vi "Adjust Text to Fit Rectangle.vi"(0 "VI Name":string, 5 "Number of Rows":i32, 7 "Text settings":T1 {"Alignment" items=["left", "center", "right"]}) -> (4 "Text out":T4)   [LabVIEW 2021, in "Text-Based VI Icon.lvlib"]
uses:
  Text-Based VI Icon.lvlib
  API_Text.ctl
  API_Test Settings.ctl
  lv_icon/Controls/Alignment.ctl
  API_Text Colors.ctl
  LabVIEW Icon API.lvlib
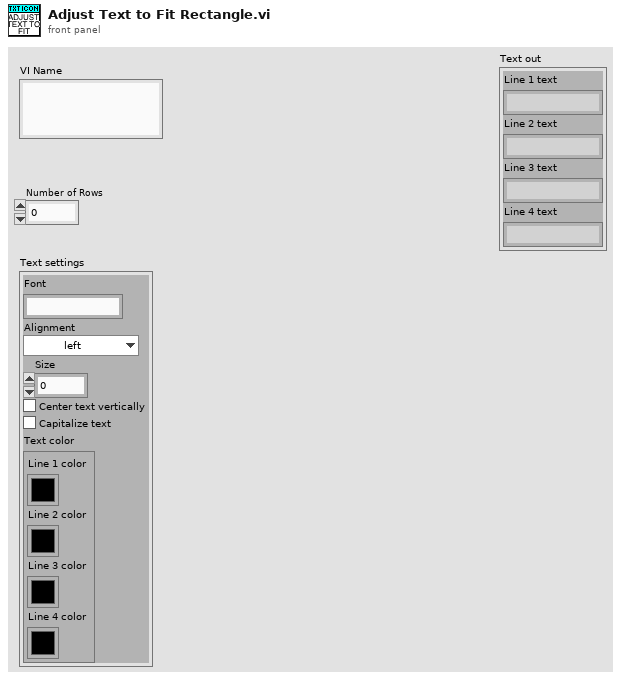
[diagram p1: front panel]
types:
  T1 = typedef "LabVIEW Icon API.lvlib/API_Test Settings.ctl" = cluster{"Font":string, "Alignment":T2, "Size":u8, "Center text":bool, "Capitalize text":bool, "Text color":T3}
  T2 = typedef "Alignment.ctl" = u16
  T3 = typedef "LabVIEW Icon API.lvlib/API_Text Colors.ctl" = cluster{"Line 1 color":u32, "Line 2 color":u32, "Line 3 color":u32, "Line 4 color":u32}
  T4 = typedef "LabVIEW Icon API.lvlib/API_Text.ctl" = cluster{"Line 1 text":string, "Line 2 text":string, "Line 3 text":string, "Line 4 text":string}
  T5 = cluster{"Font Name:":string, "Size":i16, "Strikeout?":bool, "Italic?":bool, "Underline?":bool, "Outline?":bool, "Shadow?":bool, "Bold?":bool}
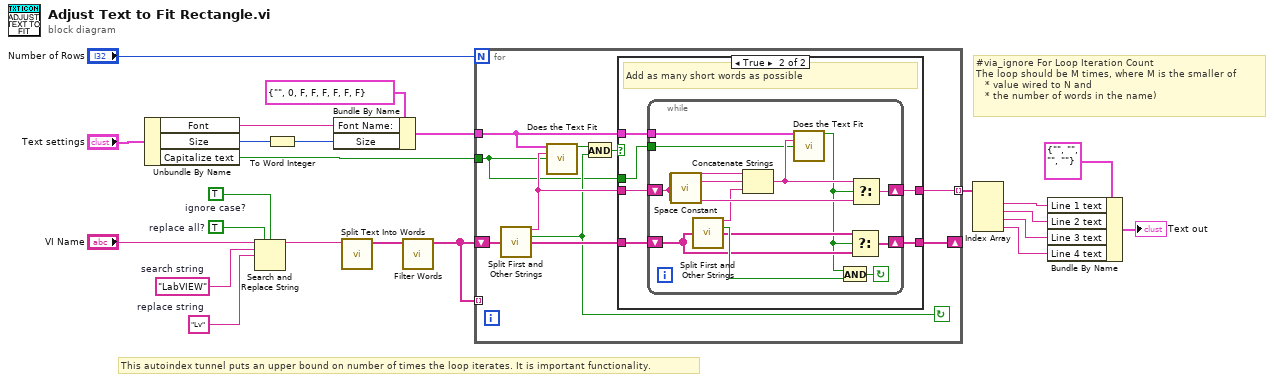
[diagram p0: block diagram]
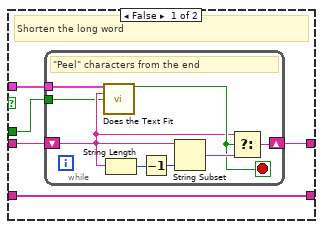
[diagram p2: hidden frame]
diagram:
  w3 = TRUE  # ignore case?
  w4 = TRUE  # replace all?
  w5 = "Lv"  # replace string
  w6 = "LabVIEW"  # search string
  # "This autoindex tunnel puts an upper bound on number of times the loop iterates. It is important functionality."
  # "#via_ignore For Loop Iteration Count\nThe loop should be M times, where M is the smaller of \n   * value wired to N and \n   * the number of words in the name)"
  n1 = Unbundle By Name("Text settings") -> ("Font"=w14:string, "Size"=w13:u8, "Capitalize text"=w9:bool)
  n2 = Search and Replace String(replace all?=w4, case sensitive?=w3, input string="VI Name", search string=w6, replace string=w5) -> (result string=w1:string)  [unwired: 3 in, 3 out]
  n3 = To Word Integer(number=w13) -> (16bit integer=w10:i16)
  n4 = Bundle By Name(cluster=T5 {"Font Name:"="", "Size"=0, "Strikeout?"=FALSE, "Italic?"=FALSE, "Underline?"=FALSE, "Outline?"=FALSE, "Shadow?"=FALSE, "Bold?"=FALSE} ("[user-specified font]"), "Font Name:"=w14, "Size"=w10) -> (w15:T5)
  n5 = call "Split Text Into Words.vi"("VI Name"=w1) -> ("Array"=w8:string[])  [unwired: 10 in]
  n6 = call "Filter Words.vi"("Array in"=w8) -> ("Array out"=w7:string[])  [unwired: 10 in]
  n7 = for {
    N: "Number of Rows" -> [_]
    tunnel: [w25] -> w18 mode=indexing
    tunnel: w15 -> [w32]
    shift-right: [w33] -> _
    shift-left: w7 -> [w29]
    tunnel: w7 -> [_] mode=indexing
    tunnel: w9 -> [w24]
    stop <- w26 continue-if-true
    n8 = call "Split First and Other Strings.vi"("Strings In"=w29) -> ("First String"=w27:string, "One or More Other Strings"=w26:bool, "Other Strings"=w28:string[])  [unwired: 12 in]
    n9 = call "Does the Text Fit.vi"("user-specified font"=w32, "token string"=w27, "Capitalize Text"=w24) -> ("Text Fits"=w31:bool)  [unwired: 12 in]
    n10 = And(x=w31, y=w26) -> (x .and. y?=w30:bool)
    n11 = case shown="True" w30 {
      tunnel: w32 -> [w35 w52]
      tunnel: w27 -> [w37 w51]
      tunnel: [w36 w50] -> w25
      tunnel: [w38 w49] -> w33
      tunnel: w28 -> [w38 w48]
      tunnel: w24 -> [w34 w47]
      frame False {
        # "Shorten the long word"
        n12 = while {
          shift-right: [w44] -> w36
          shift-left: w37 -> [w40]
          tunnel: w35 -> [w46]
          tunnel: w34 -> [w39]
          stop <- w43 stop-if-true
          # "\"Peel\" characters from the end"
          n13 = call "Does the Text Fit.vi"("user-specified font"=w46, "token string"=w40, "Capitalize Text"=w39) -> ("Text Fits"=w43:bool)  [unwired: 12 in]
          n14 = String Length(string=w40) -> (length=w42:i32)
          n15 = Decrement(x=w42) -> (x-1=w41:i32)
          n16 = String Subset(string=w40, length (rest)=w41) -> (substring=w45:string)  [unwired: 1 in]
          n17 = Select(t=w40, s=w43, f=w45) -> (s? t:f=w44:string)
        }
      }
      frame True {
        # "Add as many short words as possible"
        n18 = while {
          shift-right: [w65] -> w50
          shift-left: w51 -> [w62]
          tunnel: w52 -> [w64]
          shift-right: [w60] -> w49
          shift-left: w48 -> [w57]
          tunnel: w47 -> [w53]
          stop <- w59 continue-if-true
          n19 = call <vilib>:"Space Constant.vi"() -> ("String"=w63:string)
          n20 = call "Split First and Other Strings.vi"("Strings In"=w57) -> ("First String"=w55:string, "One or More Other Strings"=w58:bool, "Other Strings"=w56:string[])  [unwired: 12 in]
          n21 = Concatenate Strings(w62, w63, w55) -> (w61:string)
          n22 = call "Does the Text Fit.vi"("user-specified font"=w64, "token string"=w61, "Capitalize Text"=w53) -> ("Text Fits"=w54:bool)  [unwired: 12 in]
          n23 = And(x=w54, y=w58) -> (x .and. y?=w59:bool)
          n24 = Select(t=w56, s=w54, f=w57) -> (s? t:f=w60:string[])
          n25 = Select(t=w61, s=w54, f=w62) -> (s? t:f=w65:string)
        }
      }
    }
  }
  n26 = Index Array(array=w18) -> (element #1=w19:string, element #2=w20:string, element #3=w21:string, element #4=w22:string)  [unwired: 4 in]
  n27 = Bundle By Name(cluster=T4 {"Line 1 text"="", "Line 2 text"="", "Line 3 text"="", "Line 4 text"=""} ("Text out"), "Line 1 text"=w19, "Line 2 text"=w20, "Line 3 text"=w21, "Line 4 text"=w22) -> (→"Text out":T4)
